vi "test.vi"(8 "error in (no error)":errorcluster, 11 "Instrument.LN2 in":refnum<class "Instrument.LN2.lvclass">) -> (0 "error out":errorcluster, 3 "Instrument.LN2 out":refnum<class "Instrument.LN2.lvclass">)   [LabVIEW 2019, in "Instrument.LN2.lvclass"]
uses:
  Instrument.LN2.lvclass
  C:/Program Files (x86)/National Instruments/LabVIEW 2019/user.lib/LevyLab/Instrument Framework/SMOs/Instrument/Instrument.lvclass
  <userlib>/LevyLab/Instrument Framework/SMOs/Instrument/Instrument.lvclass/Instrument.ctl
  <userlib>/LevyLab/Instrument Framework/SMOs/Instrument/Instrument.lvclass
panel:
  in  "VISA resource name":refnum<visa-resource-name>
  out "Weight (kg)":dbl
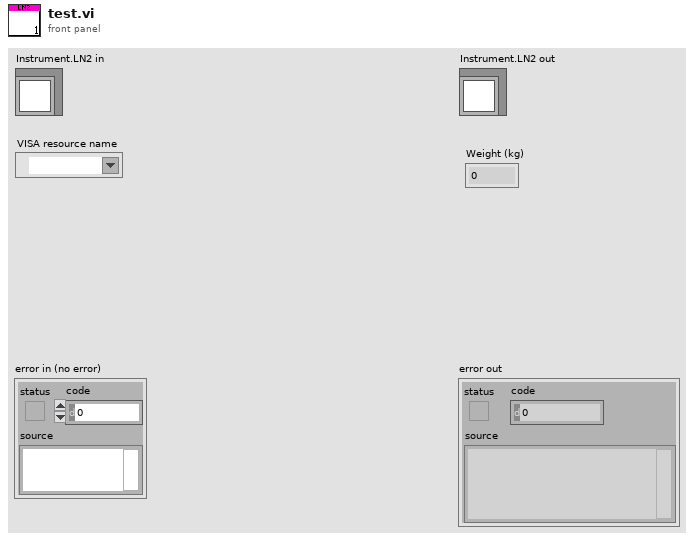
[diagram p1: front panel]
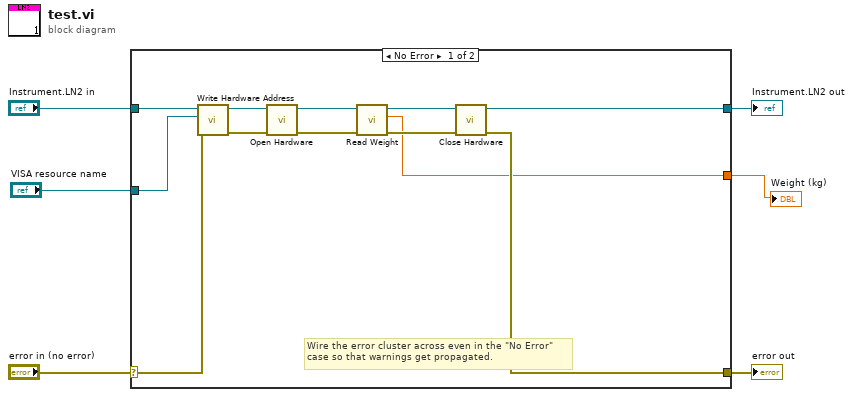
[diagram p0: block diagram]
diagram:
  n1 = case shown="No Error" "error in (no error)" {
    selector: "error in (no error)" -> [w14 w20]
    tunnel: [w17 w20] -> w5
    tunnel: [w18 w19] -> w3
    tunnel: "Instrument.LN2 in" -> [w15 w19]
    tunnel: [w7 _] -> w2
    tunnel: "VISA resource name" -> [w12 _]
    frame No Error {
      # "Wire the error cluster across even in the \"No Error\"\ncase so that warnings get propagated."
      n2 = call <userlib>:"Write Hardware Address.vi"("error in (no error)"=w14, "Address"=w12, "Instrument in"=w15) -> ("error out"=w13:errorcluster, "Instrument out"=w16:refnum<class "Instrument.LN2.lvclass">)  [unwired: 7 in]
      n3 = call-dynamic "Open Hardware.vi"("error in (no error)"=w13, "Instrument.Template in"=w16) -> ("error out"=w10:errorcluster, "Instrument.Template out"=w11:refnum<class "Instrument.LN2.lvclass">)  [unwired: 8 in]
      n4 = call "Read Weight.vi"("error in (no error)"=w10, "Instrument.LN2 in"=w11) -> ("error out"=w9:errorcluster, "Weight"=w7:dbl, "Instrument.LN2 out"=w8:refnum<class "Instrument.LN2.lvclass">)  [unwired: 7 in]
      n5 = call-dynamic "Close Hardware.vi"("error in (no error)"=w9, "Instrument.Template in"=w8) -> ("error out"=w17:errorcluster, "Instrument.Template out"=w18:refnum<class "Instrument.LN2.lvclass">)  [unwired: 8 in]
    }
    frame Error {
    }
  }
  "error out" <- w5
  "Instrument.LN2 out" <- w3
  "Weight (kg)" <- w2
